vi "VI Tree.vi"   [LabVIEW 2016, in "Control de MaP.lvlib"]
doc: "This is the instrument driver for the <INSTRUMENT NAME>. The VI Tree displays all the user-callable VIs of the instrument driver in an organized table."
uses:
  <instrlib>/Control de MaP/Control de MaP.lvlib
panel:
  # "(c) 2007 <Enter Company Name Here>.  ALL RIGHTS RESERVED."
  # "SEE DIAGRAM\nFOR VI TREE."
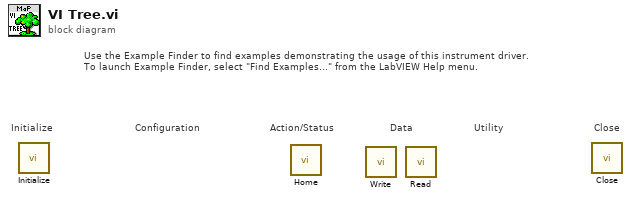
[diagram p0: block diagram]
diagram:
  # "Use the Example Finder to find examples demonstrating the usage of this instrument driver.\nTo launch Example Finder, select \"Find Examples...\" from the LabVIEW Help menu."
  # "Configuration"
  # "Utility"
  # "Data"
  # "Action/Status"
  # "Close"
  # "Initialize"
  n1 = call <instrlib>:"Initialize.vi"() -> ()  [unwired: 10 in, 2 out]
  n2 = call <instrlib>:"Home.vi"() -> ()  [unwired: 12 in]
  n3 = call <instrlib>:"Write.vi"() -> ()  [unwired: 9 in, 3 out]
  n4 = call <instrlib>:"Read.vi"() -> ()  [unwired: 9 in, 3 out]
  n5 = call <instrlib>:"Close.vi"() -> ()  [unwired: 11 in, 1 out]
